vi "SendChargingCAN.vi"(11 "CANTXQueueIn":T1) -> (3 "CANTXQueueOut":T1)   [LabVIEW 2015]
uses:
  CAN/TX Library/CAN Message Queue.ctl
  CAN/TX Library/CAN Message.ctl
  <vilib>/RioEmbeddedCAN/RioEmbeddedCAN.llb/CANFrameControl.ctl
  Global Data.vi
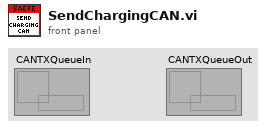
[diagram p1: front panel]
types:
  T1 = typedef "CAN Message Queue.ctl" = refnum<k33>
  T2 = typedef "CANFrameControl.ctl" = cluster{"identifier":u32, "extended?":bool, "type":u8, "payload":u8[]}
  T3 = typedef "BMS Telemetry.ctl" = cluster{"bBMSIgnition":bool, "bBMSChargerMains":bool, "bBMSFastCharge":bool, "bBMSChargerEnabled":bool, "eBMSCarState":enum16{"Off", "On, Not Charging", "Charging", "Charging Finished", "Charging Error"}, "eBMSChargingState":enum16{"Disconnected", "Pre-charging", "Main Charging", "Balancing", "Charging Finished OK", "Charging Error"}, "tBMSChargeStage":u16, "eBMSLastChargeError":enum16{"No Error", "No Cell Communication", "No Cell Communication - Non CAN Charger", "Maximum charging stage duration expired", "Cell Communication Lost during Charge", "Cannot set balancing voltage", "Cell temps too high", "No Comms so can't determine temp", "# of Cells Mismatch", "Cells Overvoltage", "Cell Protection Event occured."}, "NBMSNumCells":u8, "bBMSUnderVProtection":bool, "bBMSOverVProtection":bool, "bBMSOverTProtection":bool, "bBMSLeakageProtection":bool, "bBMSNoCellCommsError":bool, "bBMSLowVReduction":bool, "bBMSHighTReduction":bool, "VCellMin":dbl, "VCellMax":dbl, "VCellMean":dbl, "VTotal":dbl, "TCellMin":dbl, "TCellMax":dbl, "TCellMean":dbl, "VCells":cluster{"[0]":dbl, "[1]":dbl, "[2]":dbl, "[3]":dbl, "[4]":dbl, "[5]":dbl, "[6]":dbl, "[7]":dbl, "[8]":dbl, "[9]":dbl, "[10]":dbl, "[11]":dbl, "[12]":dbl, "[13]":dbl, "[14]":dbl, "[15]":dbl, "[16]":dbl, "[16] 2":dbl, "[17]":dbl, "[18]":dbl, "[19]":dbl, "[20]":dbl, "[21]":dbl, "[22]":dbl, "[23]":dbl, "[24]":dbl, "[25]":dbl, "[26]":dbl, "[27]":dbl, "[28]":dbl, "[29]":dbl, "[30]":dbl, "[31]":dbl, "[32]":dbl, "[33]":dbl, "[33] 2":dbl, "[34]":dbl, "[35]":dbl, "[36]":dbl, "[37]":dbl, "[38]":dbl, "[39]":dbl, "[40]":dbl, "[41]":dbl, "[42]":dbl, "[43]":dbl, "[44]":dbl, "[45]":dbl, "[46]":dbl, "[47]":dbl, "[48]":dbl, "[49]":dbl, "[50]":dbl, "[50] 2":dbl, "[51]":dbl, "[52] 2":dbl, "[54]":dbl, "[53]":dbl, "[55]":dbl, "[56]":dbl, "[57]":dbl, "[58]":dbl, "[59]":dbl, "[60]":dbl, "[61]":dbl, "[62]":dbl, "[63]":dbl, "[64]":dbl, "[65]":dbl, "[66]":dbl, "[67]":dbl}, "TBMSCells":cluster{"[55]":dbl, "[56]":dbl, "[57]":dbl, "[58]":dbl, "[59]":dbl, "[60]":dbl, "[61]":dbl, "[62]":dbl, "[63]":dbl, "[64]":dbl, "[65]":dbl, "[66]":dbl, "[67]":dbl, "[68]":dbl, "[69]":dbl, "[70]":dbl, "[17]":dbl, "[38]":dbl, "[39]":dbl, "[40]":dbl, "[41]":dbl, "[42]":dbl, "[43]":dbl, "[44]":dbl, "[45]":dbl, "[46]":dbl, "[47]":dbl, "[48]":dbl, "[49]":dbl, "[50]":dbl, "[51]":dbl, "[52]":dbl, "[53]":dbl, "[54]":dbl, "[21]":dbl, "[22]":dbl, "[23]":dbl, "[24]":dbl, "[25]":dbl, "[26]":dbl, "[27]":dbl, "[28]":dbl, "[29]":dbl, "[30]":dbl, "[31]":dbl, "[32]":dbl, "[33]":dbl, "[34]":dbl, "[35]":dbl, "[36]":dbl, "[37]":dbl, "[0]":dbl, "[1]":dbl, "[2]":dbl, "[3]":dbl, "[4]":dbl, "[5]":dbl, "[6]":dbl, "[7]":dbl, "[8]":dbl, "[9]":dbl, "[10]":dbl, "[11]":dbl, "[12]":dbl, "[13]":dbl, "[14]":dbl, "[15]":dbl, "[16]":dbl}, "bChargerConnected":bool, "VChargerSetpoint":dbl, "IChargerSetpoint":dbl, "VChargerActual":dbl, "IChargerActual":dbl, "BCells":cluster{"[51]":dbl, "[52]":dbl, "[53]":dbl, "[54]":dbl, "[55]":dbl, "[56]":dbl, "[57]":dbl, "[58]":dbl, "[59]":dbl, "[60]":dbl, "[61]":dbl, "[62]":dbl, "[63]":dbl, "[64]":dbl, "[65]":dbl, "[66]":dbl, "[67]":dbl, "[34]":dbl, "[35]":dbl, "[36]":dbl, "[37]":dbl, "[38]":dbl, "[39]":dbl, "[40]":dbl, "[41]":dbl, "[42]":dbl, "[43]":dbl, "[44]":dbl, "[45]":dbl, "[46]":dbl, "[47]":dbl, "[48]":dbl, "[49]":dbl, "[50]":dbl, "[17]":dbl, "[18]":dbl, "[19]":dbl, "[20]":dbl, "[21]":dbl, "[22]":dbl, "[23]":dbl, "[24]":dbl, "[25]":dbl, "[26]":dbl, "[27]":dbl, "[28]":dbl, "[29]":dbl, "[30]":dbl, "[31]":dbl, "[32]":dbl, "[33]":dbl, "[0]":dbl, "[1]":dbl, "[2]":dbl, "[3]":dbl, "[4]":dbl, "[5]":dbl, "[6]":dbl, "[7]":dbl, "[8]":dbl, "[9]":dbl, "[10]":dbl, "[11]":dbl, "[12]":dbl, "[13]":dbl, "[14]":dbl, "[15]":dbl, "[16]":dbl}, "bNewVCellMinSample":bool, "Battery Temp":cluster{"[0]":dbl, "[1]":dbl, "[2]":dbl, "[3]":dbl, "[4]":dbl, "[5]":dbl, "[6]":dbl, "[7]":dbl, "[8]":dbl, "[9]":dbl, "[10]":dbl, "[11]":dbl, "[12]":dbl, "[13]":dbl, "[14]":dbl, "[15]":dbl, "[16]":dbl, "[17]":dbl, "[18]":dbl, "[19]":dbl, "[20]":dbl, "[21]":dbl, "[22]":dbl, "[23]":dbl, "[24]":dbl, "[25]":dbl, "[26]":dbl, "[27]":dbl, "[28]":dbl, "[29]":dbl, "[30]":dbl, "[31]":dbl, "[32]":dbl, "[33]":dbl, "[34]":dbl, "[35]":dbl, "[36]":dbl, "[37]":dbl, "[38]":dbl, "[39]":dbl, "[40]":dbl, "[41]":dbl, "[42]":dbl, "[43]":dbl, "[44]":dbl, "[45]":dbl, "[46]":dbl, "[47]":dbl, "[48]":dbl, "[49]":dbl, "[50]":dbl, "[51]":dbl, "[52]":dbl, "[53]":dbl, "[54]":dbl, "[55]":dbl, "[56]":dbl, "[57]":dbl, "[58]":dbl, "[59]":dbl, "[60]":dbl, "[61]":dbl, "[62]":dbl, "[63]":dbl, "[64]":dbl, "[65]":dbl, "[66]":dbl, "[67]":dbl, "[68]":dbl, "[69]":dbl, "[70]":dbl, "[71]":dbl, "[0] 2":dbl, "[1] 2":dbl, "[2] 2":dbl, "[3] 2":dbl, "[4] 2":dbl, "[5] 2":dbl, "[6] 2":dbl, "[7] 2":dbl, "[8] 2":dbl, "[9] 2":dbl, "[10] 2":dbl, "[11] 2":dbl, "[12] 2":dbl, "[13] 2":dbl, "[14] 2":dbl, "[15] 2":dbl, "[16] 2":dbl, "[17] 2":dbl, "[18] 2":dbl, "[19] 2":dbl, "[20] 2":dbl, "[21] 2":dbl, "[22] 2":dbl, "[23] 2":dbl, "[24] 2":dbl, "[25] 2":dbl, "[26] 2":dbl, "[27] 2":dbl, "[28] 2":dbl, "[29] 2":dbl, "[30] 2":dbl, "[31] 2":dbl, "[32] 2":dbl, "[33] 2":dbl, "[34] 2":dbl, "[35] 2":dbl, "[36] 2":dbl, "[37] 2":dbl, "[38] 2":dbl, "[39] 2":dbl, "[40] 2":dbl, "[41] 2":dbl, "[42] 2":dbl, "[43] 2":dbl, "[44] 2":dbl, "[45] 2":dbl, "[46] 2":dbl, "[47] 2":dbl, "[48] 2":dbl, "[49] 2":dbl, "[50] 2":dbl, "[51] 2":dbl, "[52] 3":dbl, "[53] 2":dbl, "[54] 2":dbl, "[55] 2":dbl, "[56] 2":dbl, "[57] 2":dbl, "[58] 2":dbl, "[59] 2":dbl, "[60] 2":dbl, "[61] 2":dbl, "[62] 2":dbl, "[63] 2":dbl, "[64] 2":dbl, "[65] 2":dbl, "[66] 2":dbl, "[67] 2":dbl, "[68]2":dbl, "[69]2":dbl, "[70]2":dbl, "[71]2":dbl, "[0] 3":dbl, "[1] 3":dbl, "[2] 3":dbl, "[3] 3":dbl, "[4] 3":dbl, "[5] 3":dbl, "[6] 3":dbl, "[7] 3":dbl, "[8] 3":dbl, "[9] 3":dbl, "[10] 3":dbl, "[11] 3":dbl, "[12] 3":dbl, "[13] 3":dbl, "[14] 3":dbl, "[15] 3":dbl, "[16] 3":dbl, "[17] 3":dbl, "[18] 3":dbl, "[19] 3":dbl, "[20] 3":dbl, "[21] 3":dbl, "[22] 3":dbl, "[23] 3":dbl, "[24] 3":dbl, "[25] 3":dbl, "[26] 3":dbl, "[27] 3":dbl, "[28] 3":dbl, "[29] 3":dbl, "[30] 3":dbl, "[31] 3":dbl, "[32] 3":dbl, "[33] 3":dbl, "[34] 3":dbl, "[35] 3":dbl, "[36] 3":dbl, "[37] 3":dbl, "[38] 3":dbl, "[39] 3":dbl, "[40] 3":dbl, "[41] 3":dbl, "[42] 3":dbl, "[43] 3":dbl, "[44] 3":dbl, "[45] 3":dbl, "[46] 3":dbl, "[47] 3":dbl, "[48] 3":dbl, "[49] 3":dbl, "[50] 3":dbl, "[51] 3":dbl, "[52] 4":dbl, "[53] 3":dbl, "[54] 3":dbl, "[55] 3":dbl, "[56] 3":dbl, "[57] 3":dbl, "[58] 3":dbl, "[59] 3":dbl, "[60] 3":dbl, "[61] 3":dbl, "[62] 3":dbl, "[63] 3":dbl, "[64] 3":dbl, "[65] 3":dbl, "[66] 3":dbl, "[67] 3":dbl, "[68]3":dbl, "[69]3":dbl, "[70]3":dbl, "[71]3":dbl, "[4] 4":dbl, "[5] 4":dbl, "[6] 4":dbl, "[7] 4":dbl, "[8] 4":dbl, "[9] 4":dbl, "[10] 4":dbl, "[11] 4":dbl, "[12] 4":dbl, "[13] 4":dbl, "[14] 4":dbl, "[15] 4":dbl, "[16] 4":dbl, "[17] 4":dbl, "[18] 4":dbl, "[19] 4":dbl, "[20] 4":dbl, "[21] 4":dbl, "[22] 4":dbl, "[23] 4":dbl, "[24] 4":dbl, "[25] 4":dbl, "[26] 4":dbl, "[27] 4":dbl, "[28] 4":dbl, "[29] 4":dbl, "[30] 4":dbl, "[31] 4":dbl, "[32] 4":dbl, "[33] 4":dbl, "[17] 9":dbl, "[0] 9":dbl, "[51] 8":dbl, "[34] 8":dbl, "[17] 8":dbl, "[0] 8":dbl, "[34] 4":dbl, "[35] 4":dbl, "[36] 4":dbl, "[37] 4":dbl, "[38] 4":dbl, "[39] 4":dbl, "[40] 4":dbl, "[41] 4":dbl, "[42] 4":dbl, "[43] 4":dbl, "[44] 4":dbl, "[45] 4":dbl, "[46] 4":dbl, "[47] 4":dbl, "[48] 4":dbl, "[49] 4":dbl, "[50] 4":dbl, "[34] 9":dbl, "[51] 4":dbl, "[52] 5":dbl, "[53] 4":dbl, "[54] 4":dbl, "[55] 4":dbl, "[56] 4":dbl, "[57] 4":dbl, "[58] 4":dbl, "[59] 4":dbl, "[60] 4":dbl, "[61] 4":dbl, "[62] 4":dbl, "[63] 4":dbl, "[64] 4":dbl, "[65] 4":dbl, "[66] 4":dbl, "[67] 4":dbl, "[51] 9":dbl}, "TBMSMax":dbl, "TBMSMin":dbl, "TBMSMean":dbl, "bBMSIntRes":bool}
  T4 = enum16{"Disconnected", "Pre-charging", "Main Charging", "Balancing", "Charging Finished OK", "Charging Error"}
  T5 = enum16{"No Error", "No Cell Communication", "No Cell Communication - Non CAN Charger", "Maximum charging stage duration expired", "Cell Communication Lost during Charge", "Cannot set balancing voltage", "Cell temps too high", "No Comms so can't determine temp", "# of Cells Mismatch", "Cells Overvoltage", "Cell Protection Event occured."}
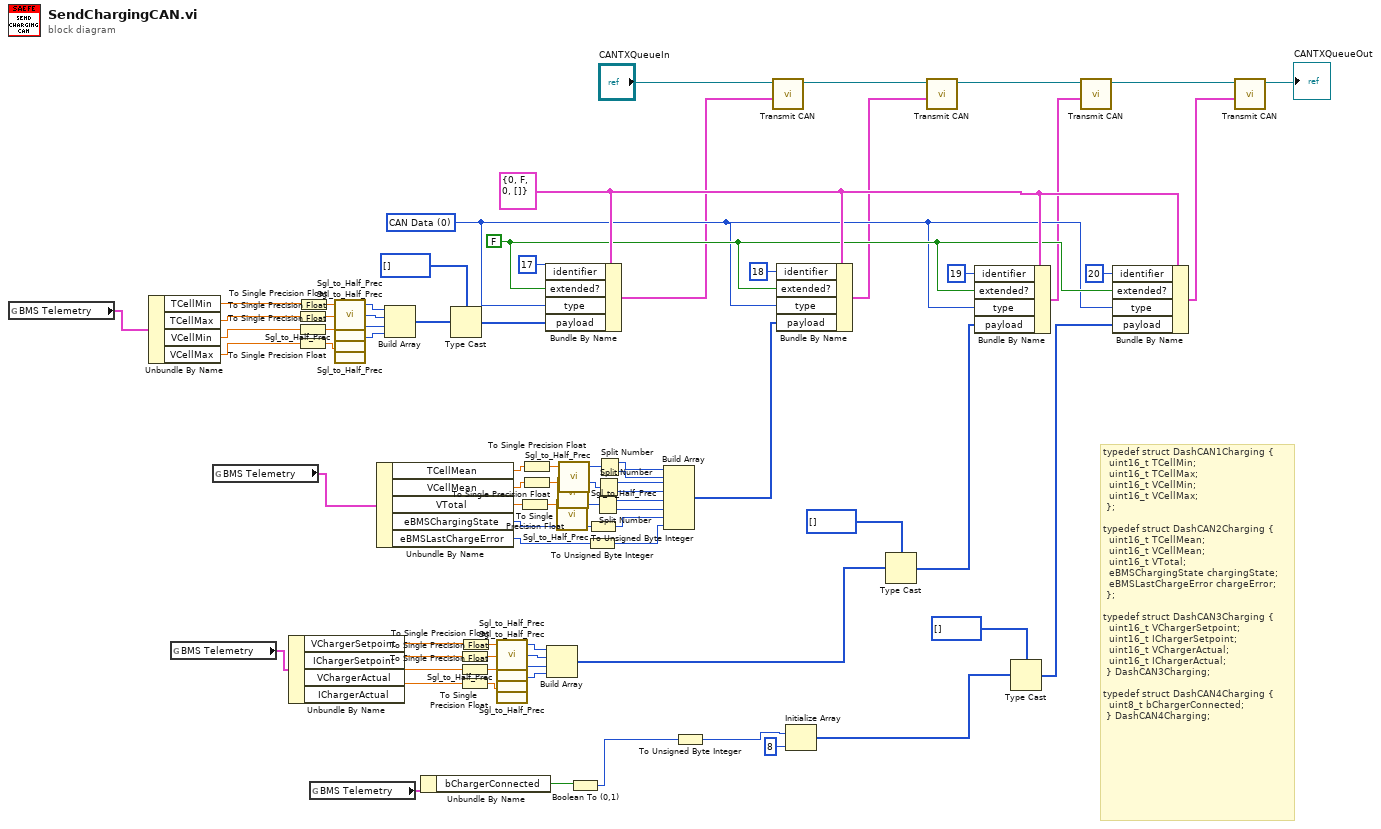
[diagram p0: block diagram]
diagram:
  w34 = u8 0 items=["CAN Data", "CAN Remote"] ("type")
  w36 = T2 {"identifier"=0, "extended?"=FALSE, "type"=0, "payload"=[]} ("CAN frame")
  w35 = FALSE ("extended?")
  # "typedef struct DashCAN1Charging {\n\t\tuint16_t TCellMin;\n\t\tuint16_t TCellMax;\n\t\tuint16_t VCellMin;\n\t\tuint16_t VCellMax;\n\t};\n\ntypedef struct DashCAN2Charging {\n\t\tuint16_t TCellMean;\n\t\tuint16_t VCellMean;\n\t\tuint16_t VTotal;\n\t\teBMSChargingState chargingState;\n\t\teBMSLastChargeError chargeError;\n\t};\n\ntypedef struct DashCAN3Charging {\n\t\tuint16_t VChargerSetpoint;\n\t\tuint16_t IChargerSetpoint;\n\t\tuint16_t VChargerActual;\n\t\tuint16_t IChargerActual;\n\t} DashCAN3Charging;\n\ntypedef struct DashCAN4Charging {\n\t\tuint8_t bChargerConnected;\n\t} DashCAN4Charging;"
  n1 = global read "Global Data.vi" "BMS Telemetry"() -> (w59:T3)
  n2 = Unbundle By Name(w59) -> ("TCellMin"=w58:dbl, "TCellMax"=w57:dbl, "VCellMin"=w56:dbl, "VCellMax"=w55:dbl)
  n3 = global read "Global Data.vi" "BMS Telemetry"() -> (w25:T3)
  n4 = global read "Global Data.vi" "BMS Telemetry"() -> (w52:T3)
  n5 = Unbundle By Name(w25) -> ("VChargerSetpoint"=w24:dbl, "IChargerSetpoint"=w23:dbl, "VChargerActual"=w22:dbl, "IChargerActual"=w21:dbl)
  n6 = To Single Precision Float(number=w57) -> (single precision float=w68:sgl)
  n7 = To Single Precision Float(number=w56) -> (single precision float=w66:sgl)
  n8 = To Single Precision Float(number=w55) -> (single precision float=w60:sgl)
  n9 = To Single Precision Float(number=w58) -> (single precision float=w67:sgl)
  n10 = global read "Global Data.vi" "BMS Telemetry"() -> (w16:T3)
  n11 = call "Sgl_to_Half_Prec.vi"("SGL"=w67) -> ("Half Precision Floating Point"=w72:u16)  [unwired: 4 in]
  n12 = call "Sgl_to_Half_Prec.vi"("SGL"=w68) -> ("Half Precision Floating Point"=w71:u16)  [unwired: 4 in]
  n13 = call "Sgl_to_Half_Prec.vi"("SGL"=w66) -> ("Half Precision Floating Point"=w70:u16)  [unwired: 4 in]
  n14 = call "Sgl_to_Half_Prec.vi"("SGL"=w60) -> ("Half Precision Floating Point"=w69:u16)  [unwired: 4 in]
  n15 = Unbundle By Name(w52) -> ("TCellMean"=w51:dbl, "VCellMean"=w50:dbl, "VTotal"=w49:dbl, "eBMSChargingState"=w48:T4, "eBMSLastChargeError"=w47:T5)
  n16 = Build Array(w72, w71, w70, w69) -> (w73:u16[])
  n17 = Unbundle By Name(w16) -> ("bChargerConnected"=w15:bool)
  n18 = Type Cast(type=u8[] [], x=w73) -> (*(type *) &x=w75:u8[])
  n19 = To Single Precision Float(number=w23) -> (single precision float=w29:sgl)
  n20 = To Single Precision Float(number=w22) -> (single precision float=w27:sgl)
  n21 = To Single Precision Float(number=w21) -> (single precision float=w26:sgl)
  n22 = To Single Precision Float(number=w24) -> (single precision float=w28:sgl)
  n23 = call "Sgl_to_Half_Prec.vi"("SGL"=w28) -> ("Half Precision Floating Point"=w33:u16)  [unwired: 4 in]
  n24 = call "Sgl_to_Half_Prec.vi"("SGL"=w29) -> ("Half Precision Floating Point"=w32:u16)  [unwired: 4 in]
  n25 = call "Sgl_to_Half_Prec.vi"("SGL"=w27) -> ("Half Precision Floating Point"=w31:u16)  [unwired: 4 in]
  n26 = call "Sgl_to_Half_Prec.vi"("SGL"=w26) -> ("Half Precision Floating Point"=w30:u16)  [unwired: 4 in]
  n27 = To Single Precision Float(number=w49) -> (single precision float=w54:sgl)
  n28 = To Single Precision Float(number=w51) -> (single precision float=w65:sgl)
  n29 = To Single Precision Float(number=w50) -> (single precision float=w64:sgl)
  n30 = Bundle By Name(cluster=w36, "identifier"=u32 17, "extended?"=w35, "type"=w34, "payload"=w75) -> (w9:T2)
  n31 = Build Array(w33, w32, w31, w30) -> (w20:u16[])
  n32 = call "Sgl_to_Half_Prec.vi"("SGL"=w54) -> ("Half Precision Floating Point"=w53:u16)  [unwired: 4 in]
  n33 = call "Sgl_to_Half_Prec.vi"("SGL"=w64) -> ("Half Precision Floating Point"=w63:u16)  [unwired: 4 in]
  n34 = call "Sgl_to_Half_Prec.vi"("SGL"=w65) -> ("Half Precision Floating Point"=w62:u16)  [unwired: 4 in]
  n35 = Boolean To (0,1)(Boolean=w15) -> (0, 1=w11:i16)
  n36 = To Unsigned Byte Integer(number=w47) -> (unsigned 8bit integer=w39:u8)
  n37 = To Unsigned Byte Integer(number=w48) -> (unsigned 8bit integer=w40:u8)
  n38 = Split Number(x=w53) -> (hi(x)=w42:u8, lo(x)=w41:u8)
  n39 = Split Number(x=w63) -> (hi(x)=w44:u8, lo(x)=w43:u8)
  n40 = Split Number(x=w62) -> (hi(x)=w46:u8, lo(x)=w45:u8)
  n41 = Build Array(w46, w45, w44, w43, w42, w41, w40, w39) -> (w61:u8[])
  n42 = To Unsigned Byte Integer(number=w11) -> (unsigned 8bit integer=w10:u8)
  n43 = call "Transmit CAN.vi"("CAN Queue"="CANTXQueueIn", "CAN frame"=w9) -> ("CAN Queue Out"=w5:T1)  [unwired: 8 in]
  n44 = Bundle By Name(cluster=w36, "identifier"=u32 18, "extended?"=w35, "type"=w34, "payload"=w61) -> (w8:T2)
  n45 = Initialize Array(w10, 8 ("dimension size")) -> (w13:u8[])
  n46 = Type Cast(type=u8[] [], x=w20) -> (*(type *) &x=w18:u8[])
  n47 = call "Transmit CAN.vi"("CAN Queue"=w5, "CAN frame"=w8) -> ("CAN Queue Out"=w4:T1)  [unwired: 8 in]
  n48 = Bundle By Name(cluster=w36, "identifier"=u32 19, "extended?"=w35, "type"=w34, "payload"=w18) -> (w7:T2)
  n49 = Type Cast(type=u8[] [], x=w13) -> (*(type *) &x=w12:u8[])
  n50 = call "Transmit CAN.vi"("CAN Queue"=w4, "CAN frame"=w7) -> ("CAN Queue Out"=w3:T1)  [unwired: 8 in]
  n51 = Bundle By Name(cluster=w36, "identifier"=u32 20, "extended?"=w35, "type"=w34, "payload"=w12) -> (w6:T2)
  n52 = call "Transmit CAN.vi"("CAN Queue"=w3, "CAN frame"=w6) -> ("CAN Queue Out"=→"CANTXQueueOut":T1)  [unwired: 8 in]
